vi "Open.vi"(8 "error in (no error)":errorcluster, 11 "MelsecTCP in":refnum<class "Inovance5UTcp.lvclass">) -> (0 "error out":errorcluster, 2 "IsSuccess":bool, 3 "MelsecTCP out":refnum<class "Inovance5UTcp.lvclass">)   [LabVIEW 2020, in "HslCommunication.lvlib" / "Inovance5UTcp.lvclass"]
uses:
  Inovance5UTcp.lvclass
  C:/Users/Fred Guo/Desktop/API_Salcomp_CMES/Libraries/HslCommunication/HslCommunication.dll
  HslCommunication.dll
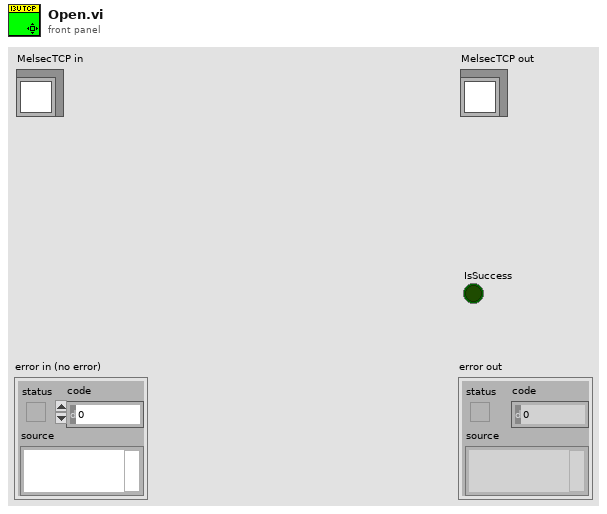
[diagram p1: front panel]
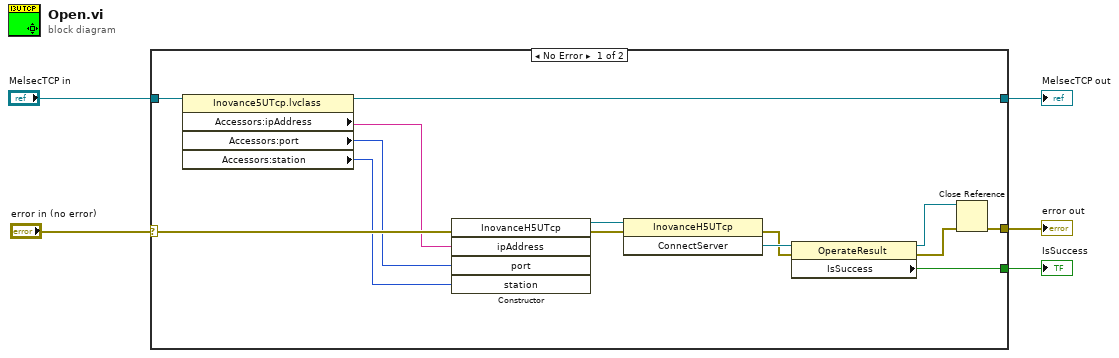
[diagram p0: block diagram]
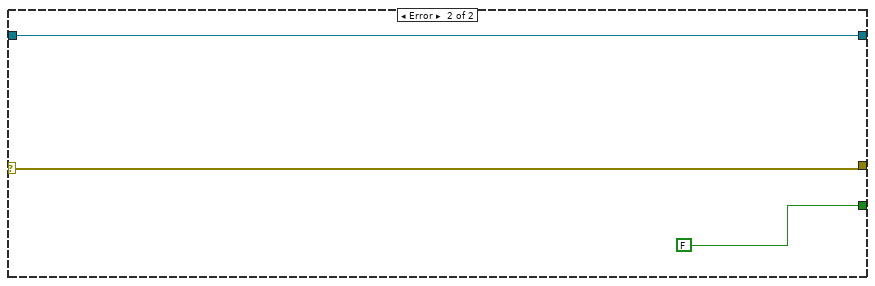
[diagram p2: hidden frame]
diagram:
  n1 = case shown="No Error" "error in (no error)" {
    selector: "error in (no error)" -> [w9 w22]
    tunnel: "MelsecTCP in" -> [w19 w21]
    tunnel: [w14 w22] -> w4
    tunnel: [w13 w21] -> w2
    tunnel: [w12 FALSE ("IsSuccess")] -> w1
    frame No Error {
      n2 = property class="Inovance5UTcp.lvclass"(reference=w19) -> (reference out=w13:refnum<class "Inovance5UTcp.lvclass">, "Accessors:ipAddress"=w8:string, "Accessors:port"=w7:i32, "Accessors:station"=w6:u8)  [unwired: 1 in, 1 out]
      n3 = constructor class="InovanceH5UTcp"(error in=w9, "ipAddress"=w8, "port"=w7, "station"=w6) -> (reference out=w11:refnum<k24>, error out=w10:errorcluster)  [unwired: 2 in, 4 out]
      n4 = invoke class="InovanceH5UTcp" method="ConnectServer"(reference=w11, error in=w10) -> (error out=w16:errorcluster, "ConnectServer"=w18:refnum<k24>)  [unwired: 1 in, 1 out]
      n5 = property class="OperateResult"(reference=w18, error in=w16) -> (reference out=w17:refnum<k24>, error out=w15:errorcluster, "IsSuccess"=w12:bool)
      n6 = Close Reference(reference=w17, error in (no error)=w15) -> (error out=w14:errorcluster)
    }
    frame Error {
    }
  }
  "error out" <- w4
  "MelsecTCP out" <- w2
  "IsSuccess" <- w1
